vi "close airyscan.vi"(8 "error in (no error)":errorcluster {"code" format="%.0x"}, 11 "camera handle":u32) -> (0 "error out":errorcluster {"code" format="%.0x"})   [LabVIEW 2015]
panel:
  in  "camera handle":u32
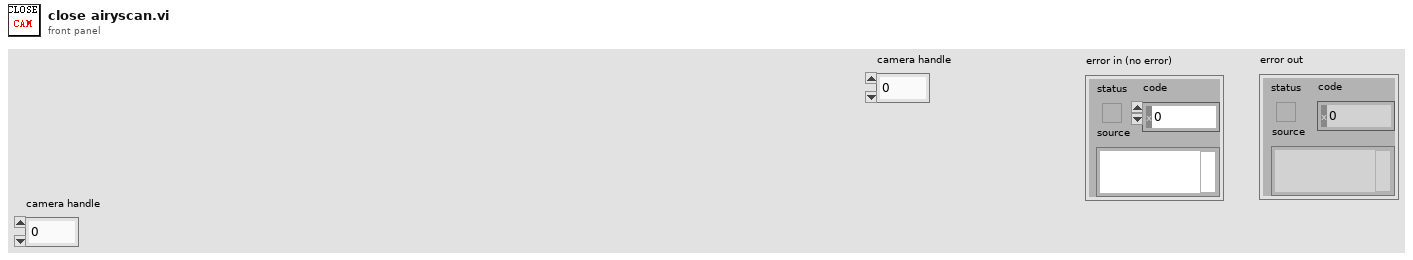
[diagram p1: front panel]
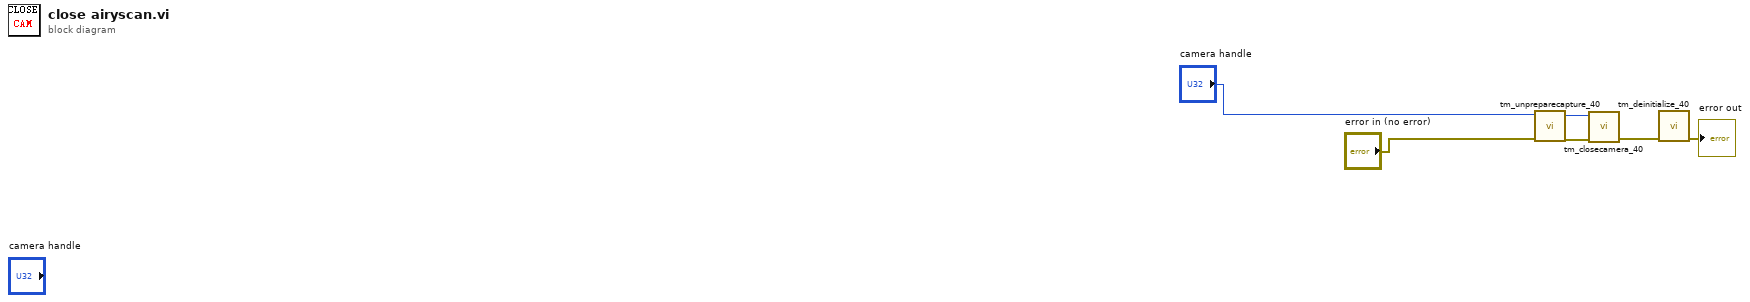
[diagram p0: block diagram]
diagram:
  n1 = call <userlib>:"tm_unpreparecapture_40.vi"("error in (no error)"="error in (no error)", "Handle in"="camera handle") -> ("error out"=w6:errorcluster, "Handle out"=w5:u32)  [unwired: 8 in]
  n2 = call <userlib>:"tm_closecamera_40.vi"("error in (no error)"=w6, "Handle in"=w5) -> ("error out"=w4:errorcluster)  [unwired: 9 in]
  n3 = call <userlib>:"tm_deinitialize_40.vi"("error in (no error)"=w4) -> ("error out"=→"error out":errorcluster)  [unwired: 10 in]
